vi "invisible button response.vi"(7 "invisible buttons":T1) -> (8 "desired move":bool[][](array[boolean]), 15 "stop loop":bool)   [LabVIEW 2019]
doc: "This subvi generates a 3x3 desired move boolean array based upon the user pushing one of the invisible buttons in the overlay cluster. It also stops the loop.\n\nPaul K Dixon\nP3600\nCSUSB Physics"
uses:
  typedefs/invisible buttons.ctl
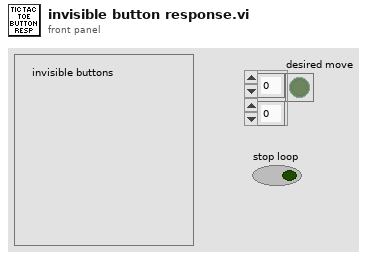
[diagram p1: front panel]
types:
  T1 = typedef "invisible buttons.ctl" = cluster{"00":bool, "01":bool, "02":bool, "10":bool, "11":bool, "12":bool, "20":bool, "21":bool, "22":bool}
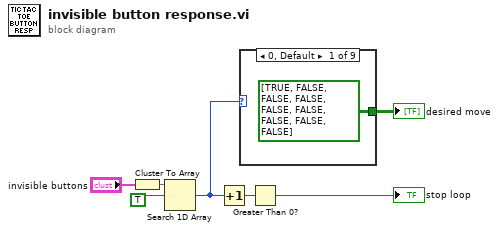
[diagram p0: block diagram]
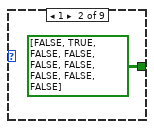
[diagram p2: hidden frame]
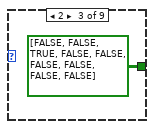
[diagram p3: hidden frame]
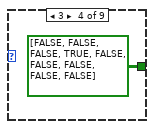
[diagram p4: hidden frame]
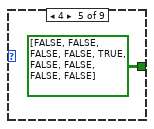
[diagram p5: hidden frame]
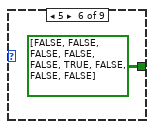
[diagram p6: hidden frame]
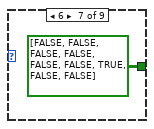
[diagram p7: hidden frame]
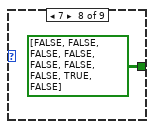
[diagram p8: hidden frame]
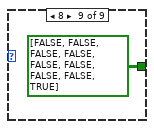
[diagram p9: hidden frame]
diagram:
  n1 = Cluster To Array(cluster="invisible buttons") -> (array=w1:bool[])
  n2 = Search 1D Array(1D array=w1, element=TRUE) -> (index of element=w6:i32)  [unwired: 1 in]
  n3 = Increment(x=w6) -> (x+1=w3:i32)
  n4 = case shown="0, Default" w6 {
    tunnel: [bool[][] [[TRUE, FALSE, FALSE], [FALSE, FALSE, FALSE], [FALSE, FALSE, FALSE]] ("desired move") bool[][] [[FALSE, TRUE, FALSE], [FALSE, FALSE, FALSE], [FALSE, FALSE, FALSE]] ("desired move") bool[][] [[FALSE, FALSE, TRUE], [FALSE, FALSE, FALSE], [FALSE, FALSE, FALSE]] ("desired move") bool[][] [[FALSE, FALSE, FALSE], [TRUE, FALSE, FALSE], [FALSE, FALSE, FALSE]] ("desired move") bool[][] [[FALSE, FALSE, FALSE], [FALSE, TRUE, FALSE], [FALSE, FALSE, FALSE]] ("desired move") bool[][] [[FALSE, FALSE, FALSE], [FALSE, FALSE, TRUE], [FALSE, FALSE, FALSE]] ("desired move") bool[][] [[FALSE, FALSE, FALSE], [FALSE, FALSE, FALSE], [TRUE, FALSE, FALSE]] ("desired move") bool[][] [[FALSE, FALSE, FALSE], [FALSE, FALSE, FALSE], [FALSE, TRUE, FALSE]] ("desired move") bool[][] [[FALSE, FALSE, FALSE], [FALSE, FALSE, FALSE], [FALSE, FALSE, TRUE]] ("desired move")] -> w7
    frame 0, Default {
    }
    frame 1 {
    }
    frame 2 {
    }
    frame 3 {
    }
    frame 4 {
    }
    frame 5 {
    }
    frame 6 {
    }
    frame 7 {
    }
    frame 8 {
    }
  }
  "desired move" <- w7
  n5 = Greater Than 0?(x=w3) -> (x > 0?=→"stop loop":bool)
